vi "GV_SetTagSelection.vi"(9 "Selection IN":T3[](array[typedef]), 11 "TAGproperties":T4 {"TAGprop"."TagFunc" format="%08x"; "TAGprop"."RangeL" format="%.2f"; "TAGprop"."RangeH" format="%.2f"}) -> (1 "SelProperties":T1[](array[typedef]), 3 "TagSelection":string[](array[string]))   [LabVIEW 2020, in "Sgraph_lib_V1.lvlib" / "Gviewer.lvclass"]
doc: "Set new TAG selection"
uses:
  Gviewer.lvclass
  DBAL/controls/DBAL_TAGprops.ctl
  DBAL/controls/DBAL_TAGpropEdit.ctl
  Common/controls/typedef_com_TagProp.ctl
  controls/EditTagOneTag.ctl
  controls/Typedef_SelProperties.ctl
  controls/Typedef_LineType.ctl
  Builds/Sgraph_lib_V1.lvlib
  DBAL/DBAL.lvclass
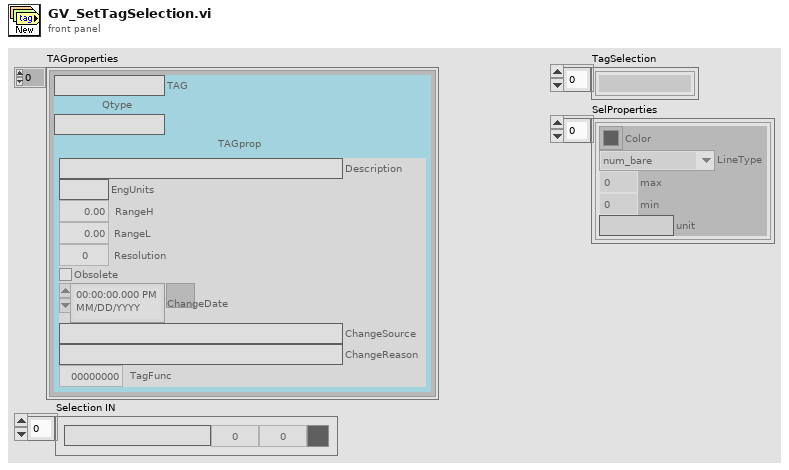
[diagram p1: front panel]
types:
  T1 = typedef "Sgraph_lib_V1.lvlib/Gviewer.lvclass/Typedef_SelProperties.ctl" = cluster{"Color":u32, "LineType":T2, "max":dbl, "min":dbl, "unit":string}
  T2 = typedef "Sgraph_lib_V1.lvlib/Gviewer.lvclass/Typedef_LineType.ctl" = enum16{"num_bare", "num_MinMax_Area", "num_MinMax_Lines", "num_MinMax_Forfor", "num_Max_Area", "num_Max_Line", "num_Max_Forfor", "num_Min_Area", "num_Min_Line", "num_Min_Fosfor", "Boolean_Line_01", "Boolean_Area_01", "Boolean_Fosfor_01", "Boolean_Line_TF", "Boolean_Area_TF", "Boolean_Fosfor_TF", "Boolean_OnOff_Line", "Boolean_OnOff_Area", "Boolean_OnOff_Fosfor", "Boolean_spare", "StringEvent_Line", "StringEvent_TimeLine"}
  T3 = typedef "Sgraph_lib_V1.lvlib/Gviewer.lvclass/EditTagOneTag.ctl" = cluster{"TAG":string, "min":dbl, "max":dbl, "Color":u32}
  T4 = typedef "Sgraph_lib_V1.lvlib/DBAL.lvclass/DBAL_TAGprops.ctl" = T5[]
  T5 = typedef "Sgraph_lib_V1.lvlib/DBAL.lvclass/DBAL_TAGpropEdit.ctl" = cluster{"TAG":string, "Qtype":string, "TAGprop":T6}
  T6 = typedef "Sgraph_lib_V1.lvlib/typedef_com_TagProp.ctl" = cluster{"Description":string, "EngUnits":string, "RangeH":dbl, "RangeL":dbl, "Resolution":i32, "Obsolete":bool, "ChangeDate":timestamp, "ChangeSource":string, "ChangeReason":string, "TagFunc":u32}
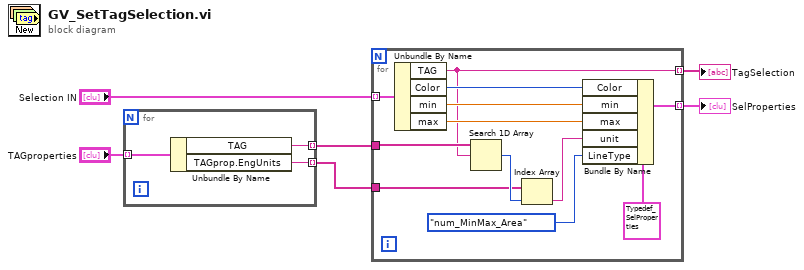
[diagram p0: block diagram]
diagram:
  n1 = for {
    tunnel: "TAGproperties" -> [w9] mode=indexing
    tunnel: [w8] -> w4 mode=indexing
    tunnel: [w7] -> w3 mode=indexing
    n2 = Unbundle By Name(w9) -> ("TAG"=w8:string, "TAGprop.EngUnits"=w7:string)
  }
  n3 = for {
    tunnel: "Selection IN" -> [w21] mode=indexing
    tunnel: [w13] -> w1 mode=indexing
    tunnel: [w16] -> w2 mode=indexing
    tunnel: w4 -> [w14]
    tunnel: w3 -> [w11]
    n4 = Unbundle By Name(w21) -> ("TAG"=w13:string, "Color"=w19:u32, "min"=w18:dbl, "max"=w17:dbl)
    n5 = Search 1D Array(1D array=w14, element=w13) -> (index of element=w12:i32)  [unwired: 1 in]
    n6 = Index Array(array=w11, index=w12) -> (element=w10:string)
    n7 = Bundle By Name(cluster=T1 {"Color"=0, "LineType"=enum."num_bare", "max"=0.0, "min"=0.0, "unit"=""} ("SelProperties"), "Color"=w19, "min"=w18, "max"=w17, "unit"=w10, "LineType"=Typedef_LineType."num_MinMax_Area") -> (w16:T1)
  }
  "TagSelection" <- w1
  "SelProperties" <- w2
